vi "Serialize MFCs.vi"() -> ()   [LabVIEW 2012]
uses:
  Devices/Alicat/Alicat Controller/Alicat Controller.lvclass
  Devices/Alicat/Controls/CtlSetup.ctl
  Devices/Alicat/Controls/Gas.ctl
  Devices/Alicat/AlicatCommBank/AlicatCommBank.lvclass
  <userlib>/Serialization/Formatter/Formatter.lvclass
  <userlib>/Serialization/Formatter/Formatter.lvclass/Formatter.ctl
  Devices/Alicat/Alicat.lvclass
  Reusable/Serial IO/Serial IO.lvclass
panel:
  in  "error in":errorcluster
  out "error out":errorcluster
  out "JSON String":string
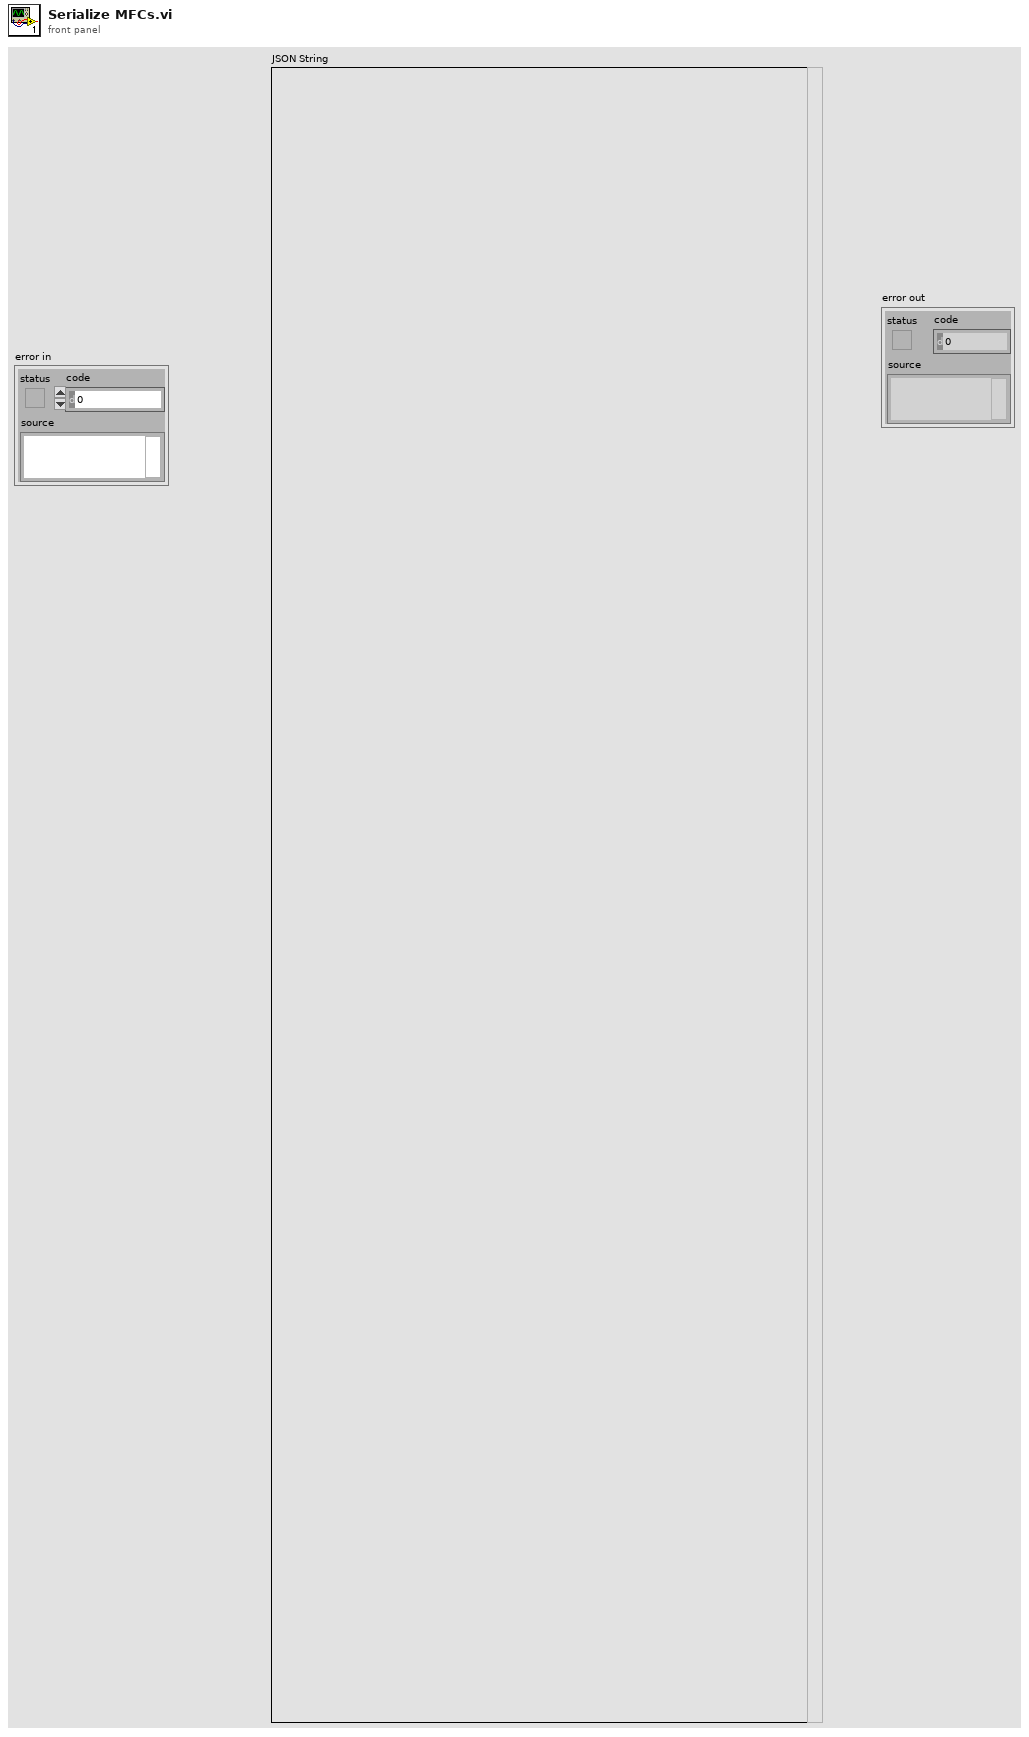
[diagram p1: front panel]
types:
  T1 = enum16{"No paths embedded", "One path with each object", "All paths with top object"}
  T2 = enum16{"open", "replace", "create", "open or create", "replace or create", "replace or create with confirmation"}
  T3 = typedef "Alicat.lvlib/Alicat.lvclass/CtlSetup.ctl" = cluster{"Name":string, "Address":string, "fullScale":dbl, "Gas":T4}
  T4 = typedef "Alicat.lvlib/Alicat.lvclass/Gas.ctl" = enum16{"Air", "Ar", "CH4", "CO", "CO2", "C2H6", "H2", "He", "N2", "NO", "Ne", "O2", "C3H8", "n-C4H10", "C2H2", "C2H4", "i-C2H10", "Kr", "Xe"}
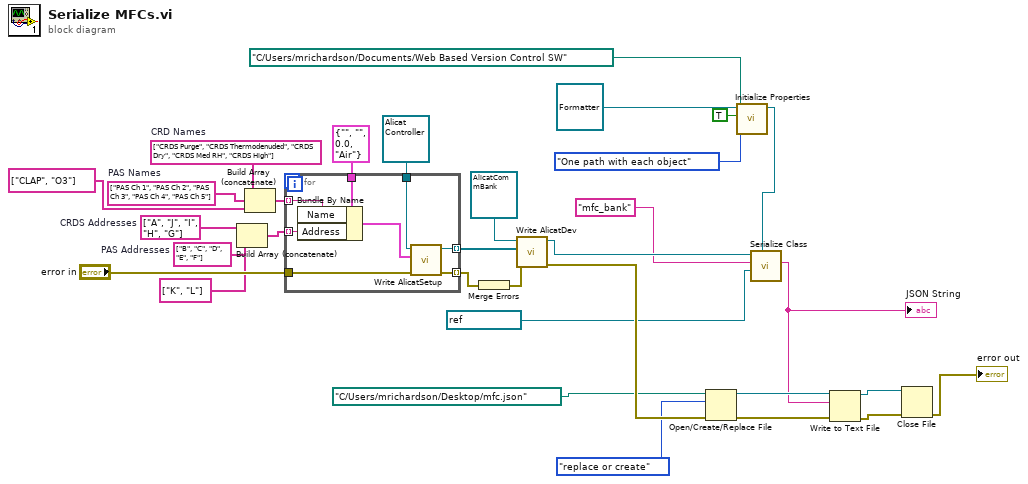
[diagram p0: block diagram]
diagram:
  w29 = string[] ["CRDS Purge", "CRDS Thermodenuded", "CRDS Dry", "CRDS Med RH", "CRDS High"]  # CRD Names
  w31 = string[] ["A", "J", "I", "H", "G"]  # CRDS Addresses
  w27 = string[] ["B", "C", "D", "E", "F"]  # PAS Addresses
  w28 = string[] ["PAS Ch 1", "PAS Ch 2", "PAS Ch 3", "PAS Ch 4", "PAS Ch 5"]  # PAS Names
  n1 = Build Array (concatenate)(w31, w27, string[] ["K", "L"] ("array")) -> (w23:string[])
  n2 = Build Array (concatenate)(w29, w28, string[] ["CLAP", "O3"] ("array")) -> (w30:string[])
  n3 = for {
    tunnel: T3 {"Name"="", "Address"="", "fullScale"=0.0, "Gas"=enum."Air"} ("AlicatSetup") -> [w38]
    tunnel: w30 -> [w37] mode=indexing
    tunnel: refnum<class "Alicat Controller.lvclass"> refnum ("Alicat") -> [w40]
    tunnel: [w39] -> w20 mode=indexing
    tunnel: w23 -> [w36] mode=indexing
    tunnel: "error in" -> [w34]
    tunnel: [w33] -> w19 mode=indexing
    n4 = Bundle By Name(cluster=w38, "Name"=w37, "Address"=w36) -> (w35:T3)
    n5 = call "Write AlicatSetup.vi"("error in"=w34, "AlicatSetup"=w35, "Alicat in"=w40) -> ("error out"=w33:errorcluster, "Alicat out"=w39:refnum<class "Alicat Controller.lvclass">)  [unwired: 7 in]
  }
  n6 = Merge Errors(w19) -> (w18:errorcluster)
  n7 = call "Write AlicatDev.vi"("error in"=w18, "AlicatDev"=w20, "AlicatCommBank in"=refnum<class "AlicatCommBank.lvclass"> refnum) -> ("error out"=w16:errorcluster, "AlicatCommBank out"=w17:refnum<class "AlicatCommBank.lvclass">)  [unwired: 7 in]
  n8 = Open/Create/Replace File(file path (use dialog)=path "C:/Users/mrichardson/Desktop/mfc.json" ("file path"), error in=w16, operation (0:open)=T2."replace or create") -> (refnum out=w14:refnum<file>, error out=w13:errorcluster)  [unwired: 3 in, 1 out]
  n9 = call <userlib>:"Initialize Properties.vi"("Absolute Path For Dynamic Loading"=path "C:/Users/mrichardson/Documents/Web Based Version Control SW", "Path Embedding"=T1."One path with each object", "Include all fields?"=TRUE, "Formatter in (Default Formatter)"=refnum<class "Formatter.lvclass"> refnum ("Formatter")) -> ("Formatter out"=w1:refnum<class "Formatter.lvclass">)  [unwired: 7 in]
  n10 = call "Serialize Class.vi"("formatter"=w1, "Port"=refnum<visa-resource-name> "MFC", "Name"="mfc_bank", "Serial IO in"=w17) -> ("JSON String"=w8:string)  [unwired: 5 in, 2 out]
  "JSON String" <- w8
  n11 = Write to Text File(file (use dialog)=w14, text=w8, error in=w13) -> (refnum out=w12:refnum<file>, error out=w11:errorcluster)  [unwired: 1 in, 1 out]
  n12 = Close File(refnum=w12, error in=w11) -> (error out=→"error out":errorcluster)  [unwired: 1 out]
